vi "4.CVT Basic Reader.vi"(8 "error in (no error)":errorcluster) -> (0 "error out":errorcluster)   [LabVIEW 2014]
uses:
  vi.lib/Q-WaveSystems/QwaveSys Raspberry Pi for LabVIEW Home-Education/QwaveSys Raspberry Pi Library.lvlib
panel:
  out "Remote Index":i32
  out "Variable Name":string="Var%d"
  out "Variable Value":dbl
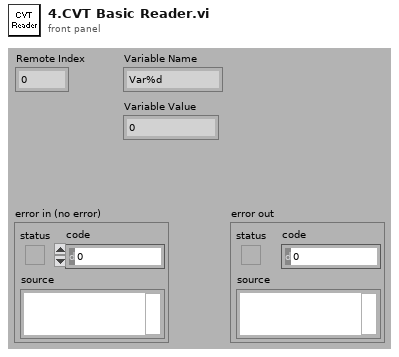
[diagram p1: front panel]
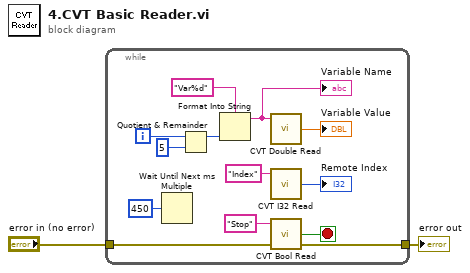
[diagram p0: block diagram]
diagram:
  n1 = while {
    tunnel: "error in (no error)" -> [w5]
    tunnel: [w4] -> w1
    i -> [w13]
    stop <- w15 stop-if-true
    n2 = Wait Until Next ms Multiple(millisecond multiple=u32 450) -> ()  [unwired: 1 out]
    n3 = Quotient & Remainder(x=w13, y=5) -> (x-y*floor(x/y)=w11:i32)  [unwired: 1 out]
    n4 = Format Into String(format string="Var%d", w11) -> (resulting string=w6:string)  [unwired: 2 in, 1 out]
    "Variable Name" <- w6
    n5 = call "CVT Double Read.vi"("Tag Name"=w6) -> ("Value"=→"Variable Value":dbl)  [unwired: 1 in, 3 out]
    n6 = call "CVT I32 Read.vi"("Tag Name"="Index") -> ("Value"=→"Remote Index":i32)  [unwired: 1 in, 3 out]
    n7 = call "CVT Bool Read.vi"("error in (no error)"=w5, "Tag Name"="Stop") -> ("error out"=w4:errorcluster, "Value"=w15:bool)  [unwired: 2 out]
  }
  "error out" <- w1
